vi "(Var)System Variables.vi"() -> ()   [LabVIEW 2020]
uses:
  Libraries/Haptic IC Class/Haptic IC/Controls/(Ctrl)IC Type.ctl
  Libraries/Haptic IC Class/Haptic IC/Haptic IC.lvclass
  Libraries/Haptic IC Class/Haptic IC/Controls/IC I2C Clock Rate.ctl
panel:
  in  "I2C Clock Rate":T1=enum."1Mhz"
  in  "Rednoah Port":refnum<visa-resource-name>
  in  "Haptic IC":refnum<class "Haptic IC.lvclass">
  out "Main VI Log Ref":refnum<vi>
  in  "IC I2C ID":u8 format="%.0x"
  in  "BD Version":u8=4
  in  "IC Type":T2=enum."DW7912"
  in  "Quit System":bool
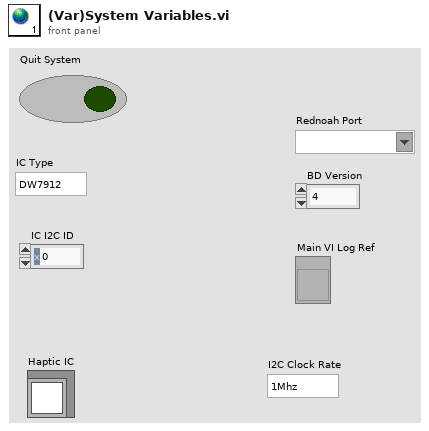
[diagram p1: front panel]
types:
  T1 = typedef "IC I2C Clock Rate.ctl" = enum8{"50khz", "100khz", "400khz", "1Mhz", "1.2Mhz"}
  T2 = typedef "Haptic IC.lvclass/(Ctrl)IC Type.ctl" = enum8{"DW7800", "DW7802", "DW7912", "DW7914"}
diagram:
